vi "test.vi"() -> ()   [LabVIEW 2012]
uses:
  <vilib>/addons/Modulation/Analog/controls/Complex Data Waveform.ctl
  <vilib>/addons/Modulation/Digital/General/MT Generate FSK System Parameters(M).vi
  <vilib>/addons/Modulation/Digital/General/MT Generate FSK Synchronization Parameters (bit array).vi
  <vilib>/Analysis/2dsp.llb/1D Cross Correlation (DBL).vi
  <vilib>/Analysis/2dsp.llb/1D Cross Correlation (CDB).vi
  <vilib>/addons/Modulation/niDMT.lvlib
  <vilib>/Analysis/NI_AALPro.lvlib
  <vilib>/addons/Modulation/niAMT.lvlib
panel:
  out "FSK error (Hz)":dbl
  out "deviation error (Hz)":dbl
  out "frequency drift (Hz)":dbl
  out "frequency offset (Hz)":dbl
  out "recovered complex waveform":T1 {"Y" format="%.3f"; "dt" format="%^.2e"; "t0" format="%.4f"}
  out "sync found index (symbols)":dbl format="%.4f"
  in  "Tab Control":T2(tab)
  out "Waveform Graph":i8[](graph)
  out "Waveform Graph 2":dbl[](graph)
  out "Waveform Graph 6":dbl[](graph)
  out "Waveform Graph 4":dbl[](graph)
  out "Waveform Graph 7":dbl[](graph)
  out "Waveform Graph 3":i8[](graph)
  out "Waveform Graph 5":dbl[](graph)
  out "Waveform Graph 8":dbl[](graph)
  out "Waveform Graph 9":dbl[](graph)
  out "ber":dbl
  out "output bit stream":i8[](array[numeric])
  out "transmitted bit sequence":i8[](array[numeric])
  out "error out":errorcluster
  out "output complex waveform":T1 caption="transmitted complex waveform" {"Y" format="%.3f"; "dt" format="%^.2e"; "t0" format="%.4f"}
  in  "FSK deviation (Hz)":dbl=150000.0 format="%.2p"
  in  "Modulation Parameters In":T3
  # "All the parameters except for the training sequence, zero pad length and # of iterations should be filled out."
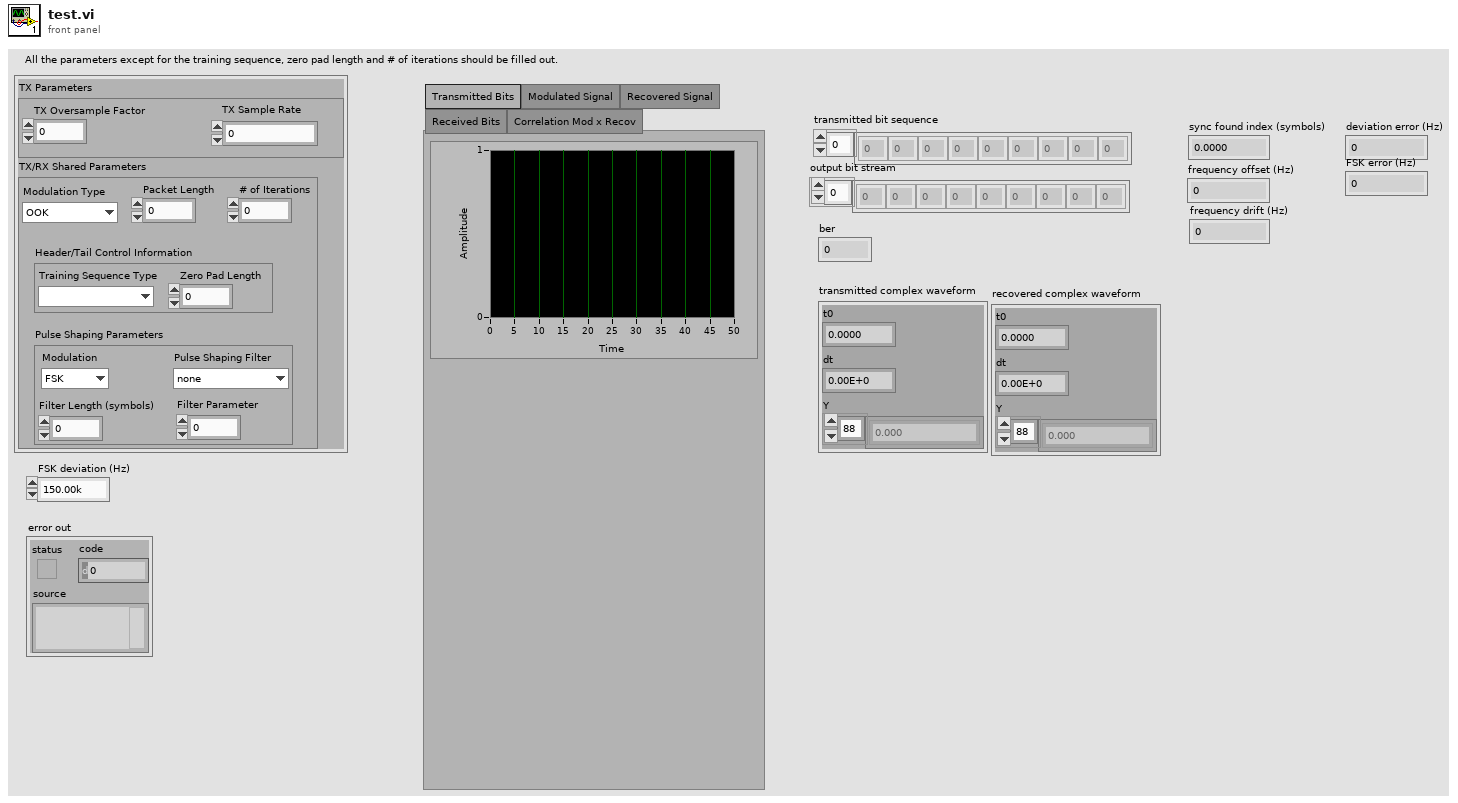
[diagram p1: front panel]
types:
  T1 = typedef "niAMT.lvlib/Complex Data Waveform.ctl" = cluster{"t0":dbl, "dt":dbl, "Y":cdb[]}
  T2 = enum32{"Transmitted Bits", "Modulated Signal", "Recovered Signal", "Received Bits", "Correlation Mod x Recov"}
  T3 = cluster{"TX Parameters":cluster{"TX Oversample Factor":i32, "TX Sample Rate":dbl}, "TX/RX Shared Parameters":cluster{"Modulation Type":enum16{"OOK", "FSK"}, "Packet Length":dbl, "# of Iterations":dbl, "Pulse Shaping Parameters":cluster{"Modulation":enum16{"FSK", "PSK", "QAM", "MSK", "PAM", "ASK", "CPM"}, "Pulse Shaping Filter":enum16{"none", "Raised Cosine", "Root Raised Cos", "Gaussian"}, "Filter Length (symbols)":i32, "Filter Parameter":dbl}, "Header/Tail Control Information":cluster{"Training Sequence Type":enum16{""}, "Zero Pad Length":dbl}}}
  T4 = enum16{"FSK", "PSK", "QAM", "MSK", "PAM", "ASK", "CPM"}
  T5 = enum16{"none", "Raised Cosine", "Root Raised Cos", "Gaussian"}
  T6 = cluster{"samples per symbol (16)":i32, "symbol map":dbl[], "symbol phase continuity":enum16{"continuous", "discontinuous"}}
  T7 = cluster{"expected sync location (symbols)":i32, "sync sequence":cdb[], "sync location uncertainty (symbols)":i32, "sync indent (symbols)":i32}
  T8 = cluster{"frequency offset (Hz)":dbl, "frequency drift (Hz)":dbl, "deviation error (Hz)":dbl, "FSK error (Hz)":dbl}
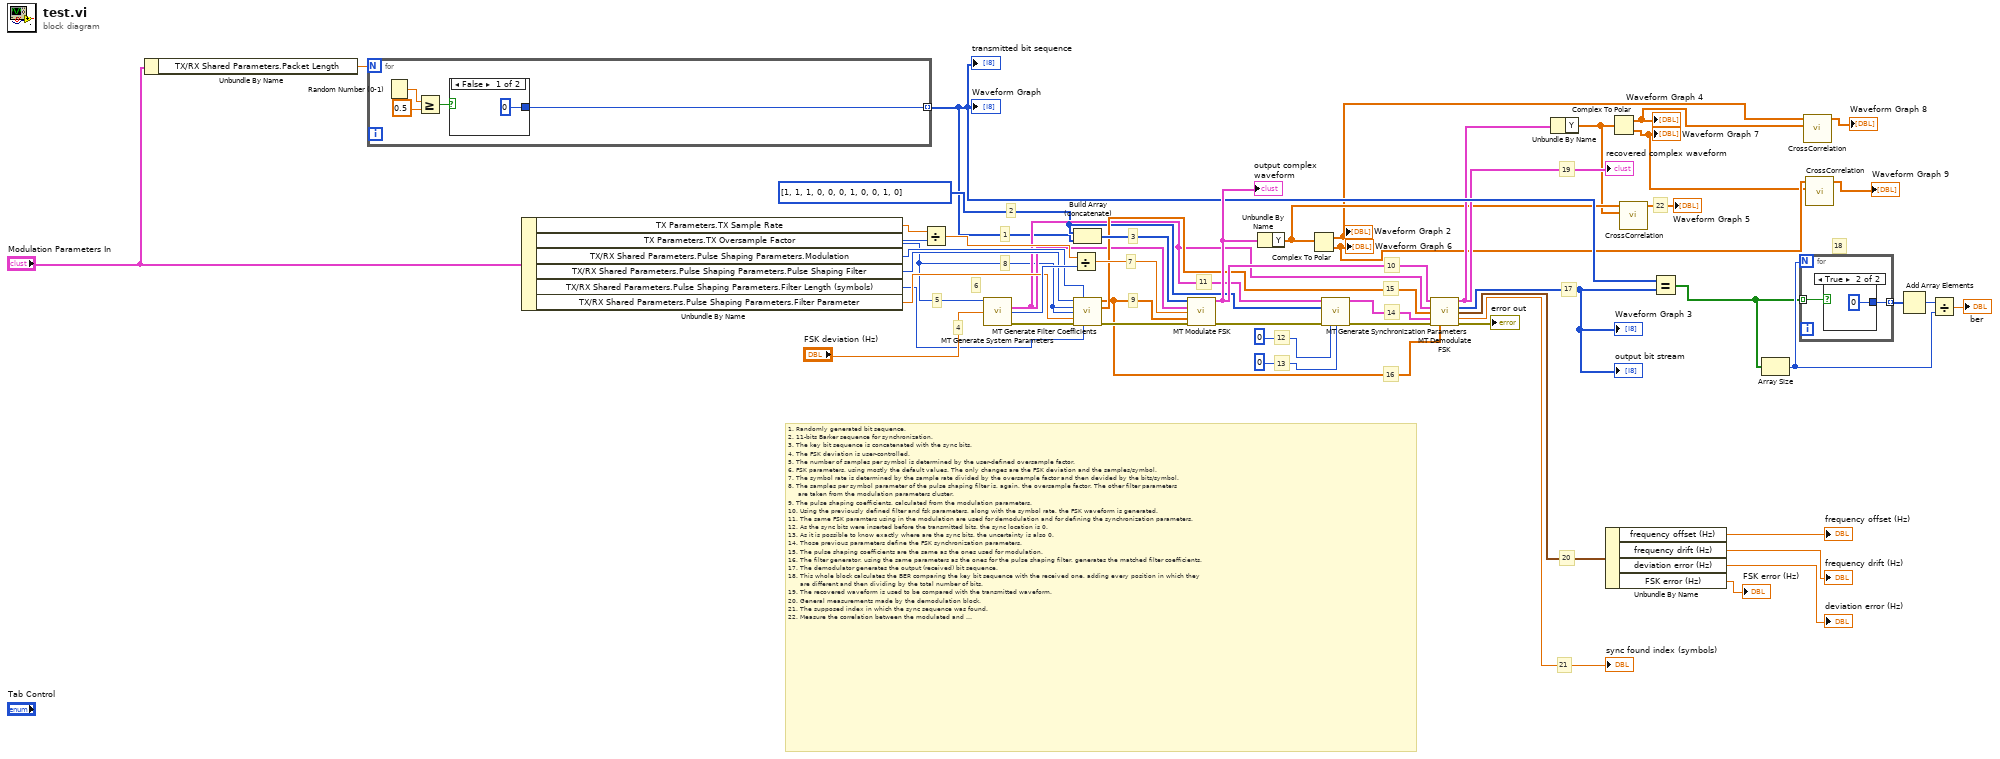
[diagram p0: block diagram]
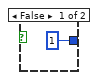
[diagram p2: hidden frame]
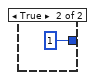
[diagram p3: hidden frame]
diagram:
  w27 = i8[] [1, 1, 1, 0, 0, 0, 1, 0, 0, 1, 0] ("sync bits")
  # "22"
  # "1. Randomly generated bit sequence.\n2. 11-bits Barker sequence for synchronization.\n3. The key bit sequence is concatenated with the sync bits.\n4. The FSK deviation is user-controlled.\n5. The number of samples per symbol is determined by the user-defined oversample factor.\n6. FSK parameters, using mostly the default values. The only changes are the FSK deviation and the samples/symbol.\n7. The symbol rate is determined by the sample rate divided by the oversample factor and then devided by the bits/symbol.\n8. The samples per symbol parameter of the pulse shaping filter is, again, the oversample factor. The other filter parameters\n     are taken from the modulation parameters cluster.\n9. The pulse shaping coefficients, calculated from the modulation parameters.\n10. Using the previously defined filter and fsk parameters, along with the symbol rate, the FSK waveform is generated.\n11. The same FSK paramters using in the modulation are used for demodulation and for defining the synchronization parameters.\n12. As the sync bits were inserted before the transmitted bits, the sync location is 0.\n13. As it is possible to know exactly where are the sync bits, the uncertainty is also 0.\n14. Those previous parameters define the FSK synchronization parameters.\n15. The pulse shaping coefficients are the same as the ones used for modulation.\n16. The filter generator, using the same parameters as the ones for the pulse shaping filter, generates the matched filter coefficients.\n17. The demodulator generates the output (received) bit sequence.\n18. This whole block calculates the BER comparing the key bit sequence with the received one, adding every position in which they\n      are different and then dividing by the total number of bits.\n19. The recovered waveform is used to be compared with the transmitted waveform.\n20. General measurements made by the demodulation block.\n21. The supposed index in which the sync sequence was found.\n22. Measure the correlation between the modulated and the recovered signals."
  # "21"
  # "20"
  # "19"
  # "18"
  # "17"
  # "16"
  # "15"
  # "14"
  # "13"
  # "12"
  # "11"
  # "10"
  # "9"
  # "8"
  # "7"
  # "6"
  # "5"
  # "4"
  # "3"
  # "2"
  # "1"
  n1 = Unbundle By Name("Modulation Parameters In") -> ("TX/RX Shared Parameters.Packet Length"=w49:dbl)
  n2 = for {
    N: w49 -> [_]
    tunnel: [w50] -> w21 mode=indexing
    n3 = Random Number (0-1)() -> (number: 0 to 1=w52:dbl)
    n4 = Greater Or Equal?(x=w52, y=0.5) -> (x >= y?=w51:bool)
    n5 = case shown="False" w51 {
      tunnel: [i8 0 i8 1] -> w50
      frame False {
      }
      frame True {
      }
    }
  }
  "Waveform Graph" <- w21
  "transmitted bit sequence" <- w21
  n6 = Unbundle By Name("Modulation Parameters In") -> ("TX Parameters.TX Sample Rate"=w41:dbl, "TX Parameters.TX Oversample Factor"=w11:i32, "TX/RX Shared Parameters.Pulse Shaping Parameters.Modulation"=w37:T4, "TX/RX Shared Parameters.Pulse Shaping Parameters.Pulse Shaping Filter"=w36:T5, "TX/RX Shared Parameters.Pulse Shaping Parameters.Filter Length (symbols)"=w33:i32, "TX/RX Shared Parameters.Pulse Shaping Parameters.Filter Parameter"=w35:dbl)
  n7 = Divide(x=w41, y=w11) -> (x/y=w40:dbl)
  n8 = call-poly <vilib>:"MT Generate System Parameters.vi"("samples per symbol (16)"=w11, "FSK deviation (Hz)"="FSK deviation (Hz)") -> ("FSK system parameters"=w28:T6, "bits per symbol"=w39:i32, "error out"=w34:errorcluster)  [unwired: 11 in]
  n9 = Divide(x=w40, y=w39) -> (x/y=w38:dbl)
  n10 = Build Array (concatenate)(w27, w21) -> (w43:i8[])
  n11 = call <vilib>:"MT Generate Filter Coefficients.vi"("pulse shaping filter (none)"=w36, "modulation type"=w37, "pulse shaping samples per symbol (16)"=w11, "matched samples per symbol (16)"=w11, "filter parameter"=w35, "error in (no error)"=w34, "filter length (symbols)"=w33) -> ("pulse shaping filter coefficients"=w29:dbl[], "matched filter coefficients"=w30:dbl[], "error out"=w32:errorcluster)  [unwired: 6 in]
  n12 = call <vilib>:"MT Modulate FSK.vi"("input bit stream"=w43, "FSK system parameters"=w28, "symbol rate (Hz)"=w38, "pulse shaping filter coefficients"=w29, "error in (no error)"=w32) -> ("output complex waveform"=w31:T1, "error out"=w26:errorcluster)  [unwired: 8 in, 1 out]
  "output complex waveform" <- w31
  n13 = Unbundle By Name(w31) -> ("Y"=w8:cdb[])
  n14 = Complex To Polar(r * e^(i*theta)=w8) -> (r=w5:dbl[], theta=w4:dbl[])
  "Waveform Graph 2" <- w5
  "Waveform Graph 6" <- w4
  n15 = call-poly <vilib>:"MT Generate Synchronization Parameters.vi"("FSK system parameters"=w28, "sync bits"=w27, "error in (no error)"=w26, "expected sync location (symbols)"=0, "sync location uncertainty (symbols)"=0) -> ("FSK synchronization parameters"=w22:T7, "error out"=w23:errorcluster)  [unwired: 9 in]
  n16 = call <vilib>:"MT Demodulate FSK.vi"("input complex waveform"=w31, "FSK system parameters"=w28, "matched filter coefficients"=w30, "synchronization parameters"=w22, "error in (no error)"=w23, "pulse shaping filter coefficients"=w29) -> ("recovered complex waveform"=w10:T1, "output bit stream"=w18:i8[], "measurements"=w17:T8, "sync found index (symbols)"=→"sync found index (symbols)":dbl, "error out"=→"error out":errorcluster)  [unwired: 5 in]
  "Waveform Graph 3" <- w18
  "output bit stream" <- w18
  "recovered complex waveform" <- w10
  n17 = Unbundle By Name(w10) -> ("Y"=w7:cdb[])
  n18 = Unbundle By Name(w17) -> ("frequency offset (Hz)"=→"frequency offset (Hz)":dbl, "frequency drift (Hz)"=→"frequency drift (Hz)":dbl, "deviation error (Hz)"=→"deviation error (Hz)":dbl, "FSK error (Hz)"=→"FSK error (Hz)":dbl)
  n19 = Complex To Polar(r * e^(i*theta)=w7) -> (r=w6:dbl[], theta=w3:dbl[])
  "Waveform Graph 4" <- w6
  "Waveform Graph 7" <- w3
  n20 = call-poly <vilib>:"CrossCorrelation.vi"("Y"=w7, "X"=w8) -> ("Rxy"=→"Waveform Graph 5":cdb[])  [unwired: 8 in, 1 out]
  n21 = Equal?(x=w21, y=w18) -> (x = y?=w20:bool[])
  n22 = Array Size(array=w20) -> (size(s)=w45:i32)
  n23 = for {
    N: w45 -> [_]
    tunnel: [w57] -> w47 mode=indexing
    tunnel: w20 -> [w56] mode=indexing
    n24 = case shown="True" w56 {
      tunnel: [1 0] -> w57
      frame False {
      }
      frame True {
      }
    }
  }
  n25 = call-poly <vilib>:"CrossCorrelation.vi"("Y"=w6, "X"=w5) -> ("Rxy"=→"Waveform Graph 8":dbl[])  [unwired: 8 in, 1 out]
  n26 = call-poly <vilib>:"CrossCorrelation.vi"("Y"=w3, "X"=w4) -> ("Rxy"=→"Waveform Graph 9":dbl[])  [unwired: 8 in, 1 out]
  n27 = Add Array Elements(numeric array=w47) -> (sum=w46:i32)
  n28 = Divide(x=w46, y=w45) -> (x/y=→"ber":dbl)
